vi "소푸틴의 뜻밖의 여정.vi"() -> ()   [LabVIEW 2019]
uses:
  <vilib>/Platform/TimedLoop/XDataNode/timing_clust.ctl
  <vilib>/Platform/TimedLoop/XDataNode/nitl_modes.ctl
  <vilib>/Platform/TimedLoop/XDataNode/wakeup.ctl
  <vilib>/FPGAPlugInAG/myRIO-1900/niLvFpga_Open_myRIO-1900.vi
  <vilib>/rvi/interface/common/dynamic/niFpgaDynamicAddResources.vi
  <vilib>/Utility/error.llb/Error Cluster From Error Code.vi
  <vilib>/rvi/errors/niLvFpgaAdjustHostInterfaceError.vi
  <vilib>/FPGAPlugInAG/Dynamic/niLvFpga_Close_Dynamic.vi
  <vilib>/Platform/TimedLoop/XDataNode/XDataNode.xnode
  <vilib>/rvi/interface/nirviOpenFPGA/nirviOpenFPGA.xnode
  FPGA Bitfiles/untitledproject2_FPGATarget_EncoderPWM(6)2_XV2oDltnHKU.lvbitx
  Encoder_PWM (6).vi
  <vilib>/rvi/interface/nirviReadWriteControl/nirviReadWriteControl.xnode
  <vilib>/rvi/interface/nirviCloseFPGA/nirviCloseFPGA.xnode
  NiFpgaLv.dll
  <vilib>/rvi/interface/Simulation/niFpgaSimulationCallBeginRW.vi
  <vilib>/Platform/TimedLoop/XDataNode/XDNodeRunTimeDep.lvlib
panel:
  out "왼불 5":bool
  out "오른불 4":bool
  out "좌회전":dbl
  out "좌회전":dbl
  out "소푸틴 왼발자취 2":dbl
  out "소푸틴 오른발자취 2":dbl
  in  "stop":bool
  out "왼불 2":bool
  out "오불":bool
  out "소푸틴 왼발자취":dbl
  out "직진 6":dbl
  out "우회전 (30도) 2":dbl
  out "직진 5":dbl
  out "우회전 2":dbl
  out "직진 4":dbl
  out "좌회전 2":dbl
  out "소푸틴 오른발자취":dbl
  in  "초음파":dbl
  in  "잿슨나노":dbl
  out "직진 3":dbl
  out "우회전 (30도)":dbl
  out "직진 2":dbl
  out "우회전":dbl
  out "직진":dbl
  out "좌회전":dbl
  out "Input L 3":dbl[](graph)
  out "Reference & Measurement_L 3":dbl[][](graph)
  in  "Ki 2":dbl
  in  "Kd 2":dbl
  in  "Kp_L":dbl
  out "Input R 2":dbl[](graph)
  out "Reference & Measurement_R 2":dbl[][](graph)
  in  "Ki":dbl
  in  "Kd":dbl
  in  "Kp_R":dbl
  out "u 7":dbl
  out "Mea 4":dbl
  out "Enc_r 2":i32
  out "R_ref":dbl
  out "u 6":dbl
  out "Mea 5":dbl
  out "Enc_r 3":i32
  out "L_ref":dbl
  out "enc":bool
  # "-----------------------------------------------장애물--------------------------------------------------------------"
  # "오른쪽"
  # "왼쪽"
  # "초음파거리 20cm 기준!!"
  # "2200   1700\n\n60    40\n\n\n40   70"
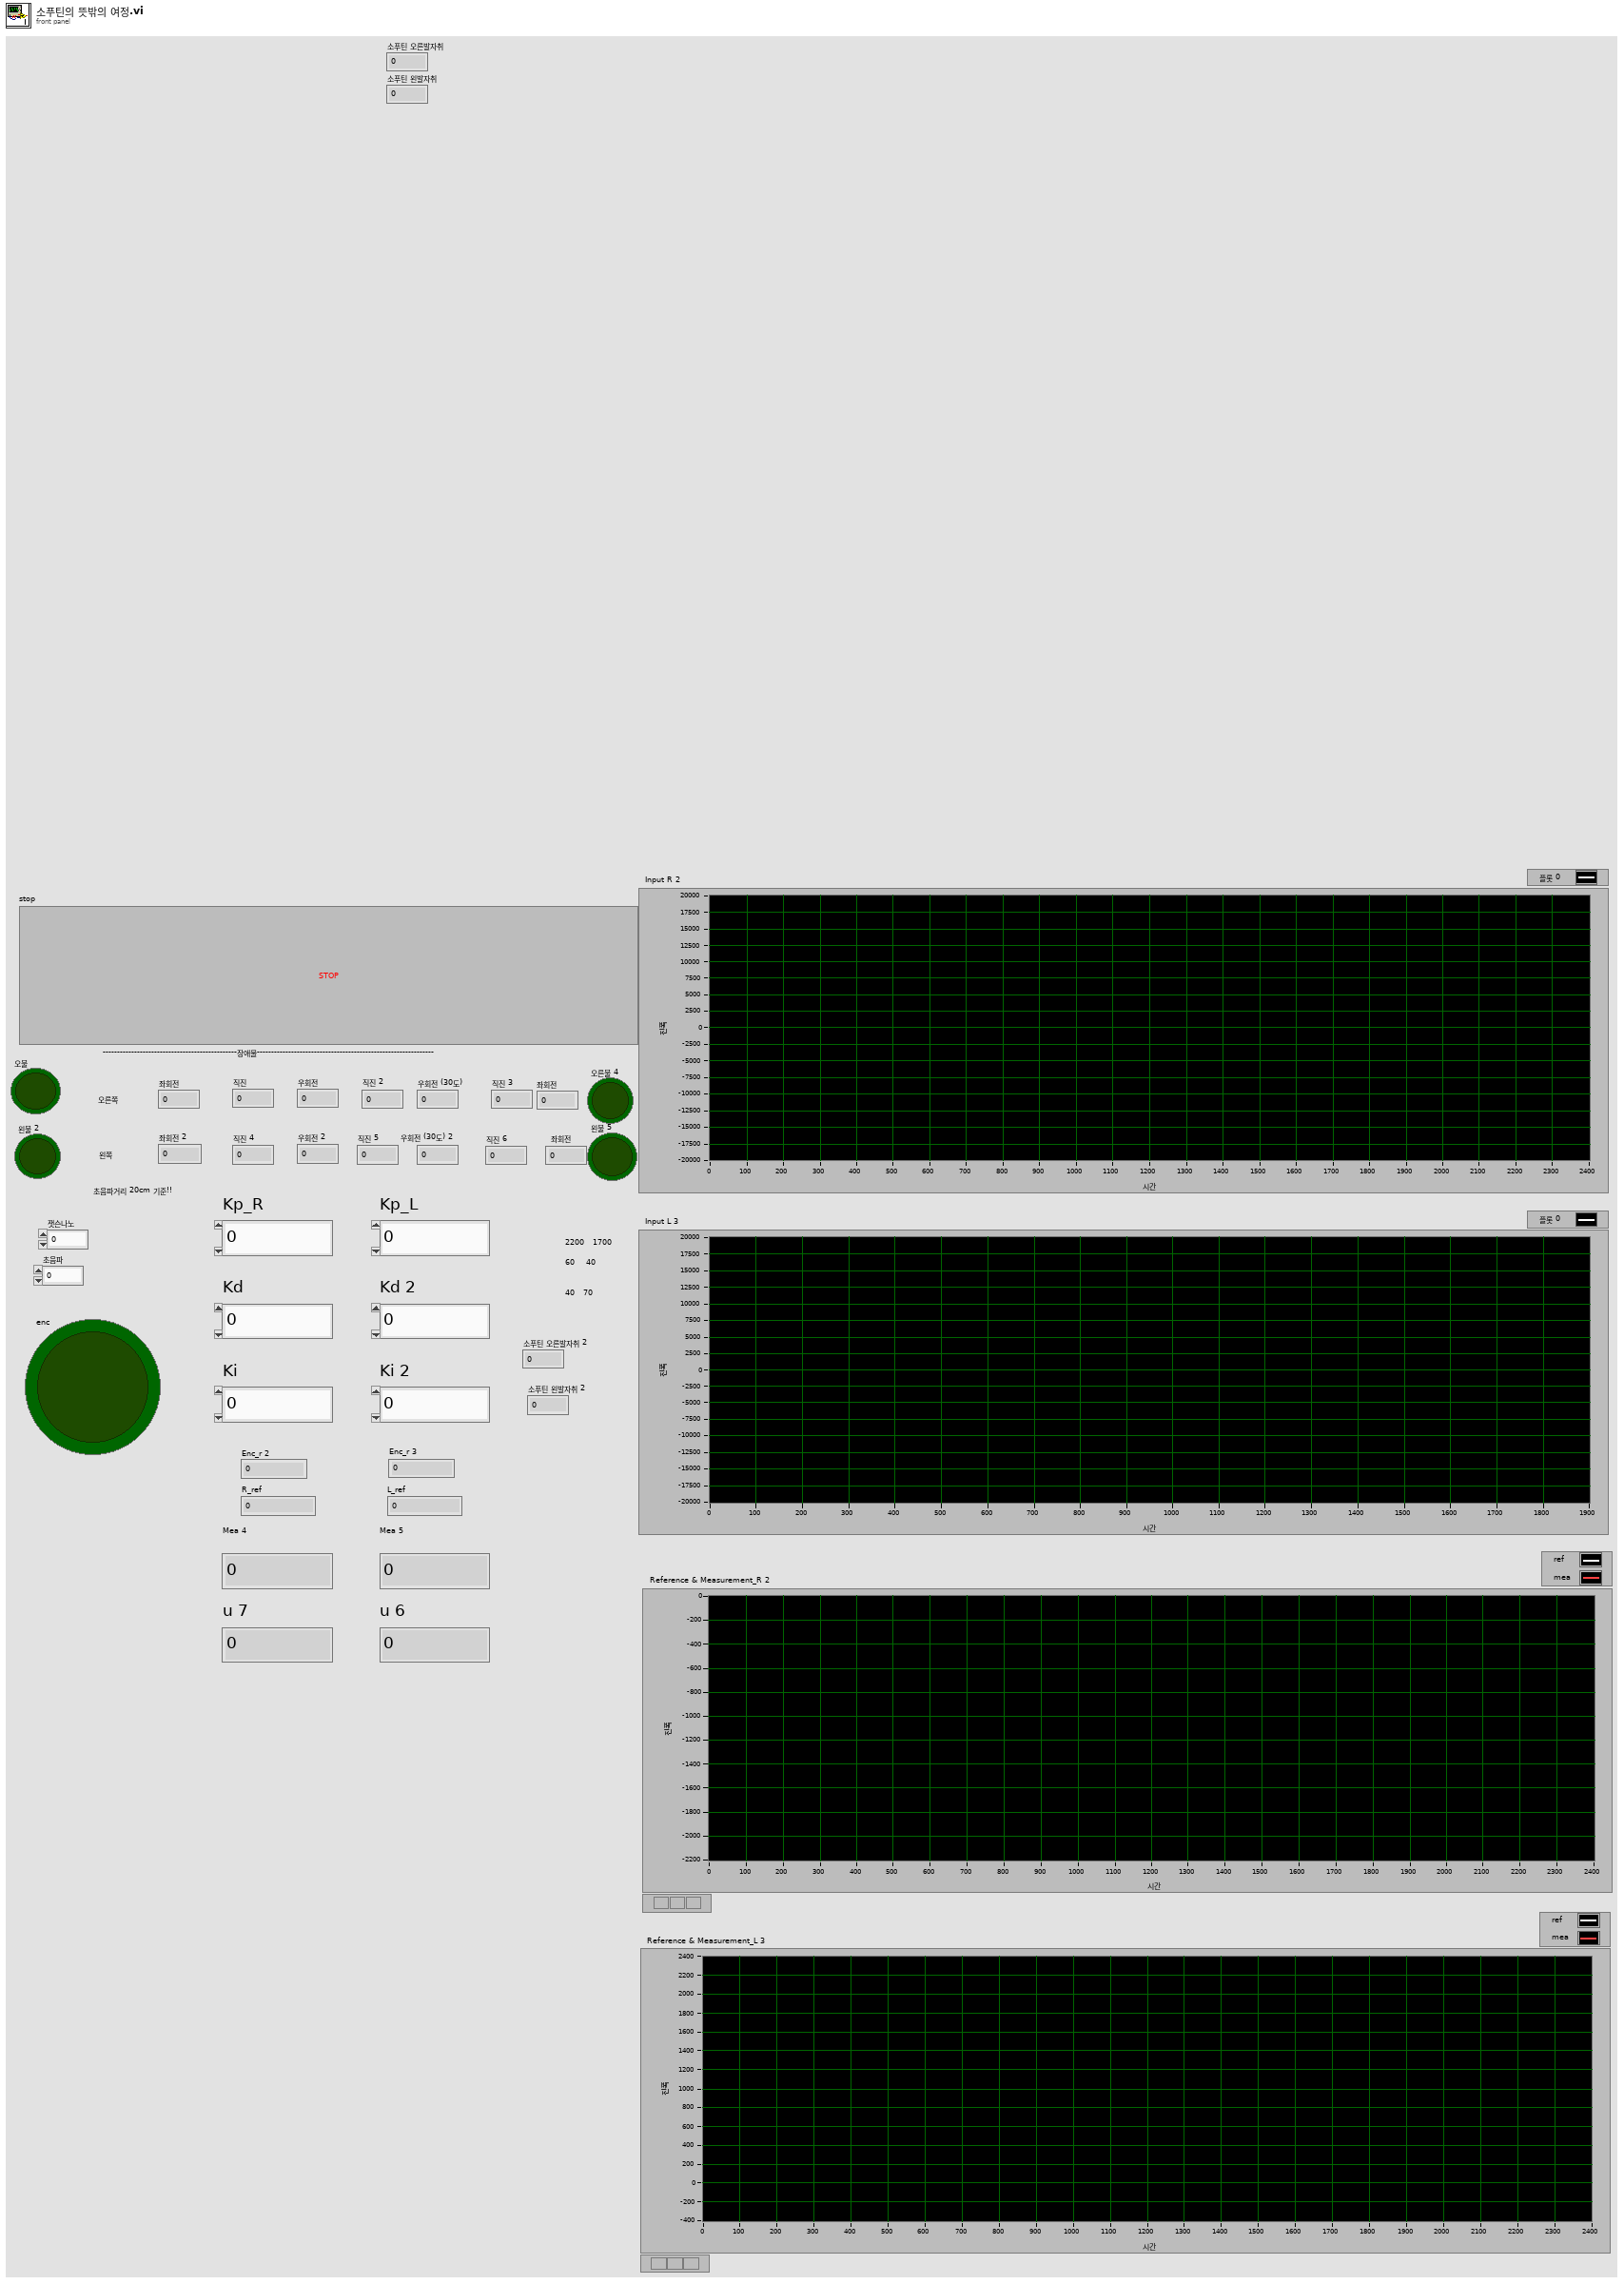
[diagram p1: front panel]
types:
  T1 = typedef "XDNodeRunTimeDep.lvlib/timing_clust.ctl" = cluster{"Expected End [f-1]":u64, "Actual End [f-1]":u64, "Finished Late? [f-1]":bool, "Expected End [i-1]":u64, "Actual End [i-1]":u64, "Finished Late? [i-1]":bool, "Expected Start [i]":u64, "Actual Start [i]":u64, "Expected Start [f]":u64, "Actual Start [f]":u64, "Source Name":string, "Structure Name":string, "Period":i64, "Deadline":i64, "Offset":i64, "Start":i64, "Priority":i32, "Timeout":i32, "Mode":T2, "Wakeup Reason":T3, "Error":errorcluster, "Source Type":string, "Secondary Source Type":string, "Global End Time":u64, "Global Start Time":u64, "Frame Duration":u64, "Iteration Duration":u64, "Assigned CPU":i32, "I/O Scan Engine Mode":u32}
  T2 = typedef "XDNodeRunTimeDep.lvlib/nitl_modes.ctl" = enum32{"No Change", "Process missed periods, maintain original phase", "Discard missed periods, maintain original phase", "Process missed periods, ignore original phase", "Discard missed periods, ignore original phase"}
  T3 = typedef "XDNodeRunTimeDep.lvlib/wakeup.ctl" = enum32{"Normal", "Aborted", "Asynchronous wakeup", "Timing source error", "Timed loop error", "Timeout"}
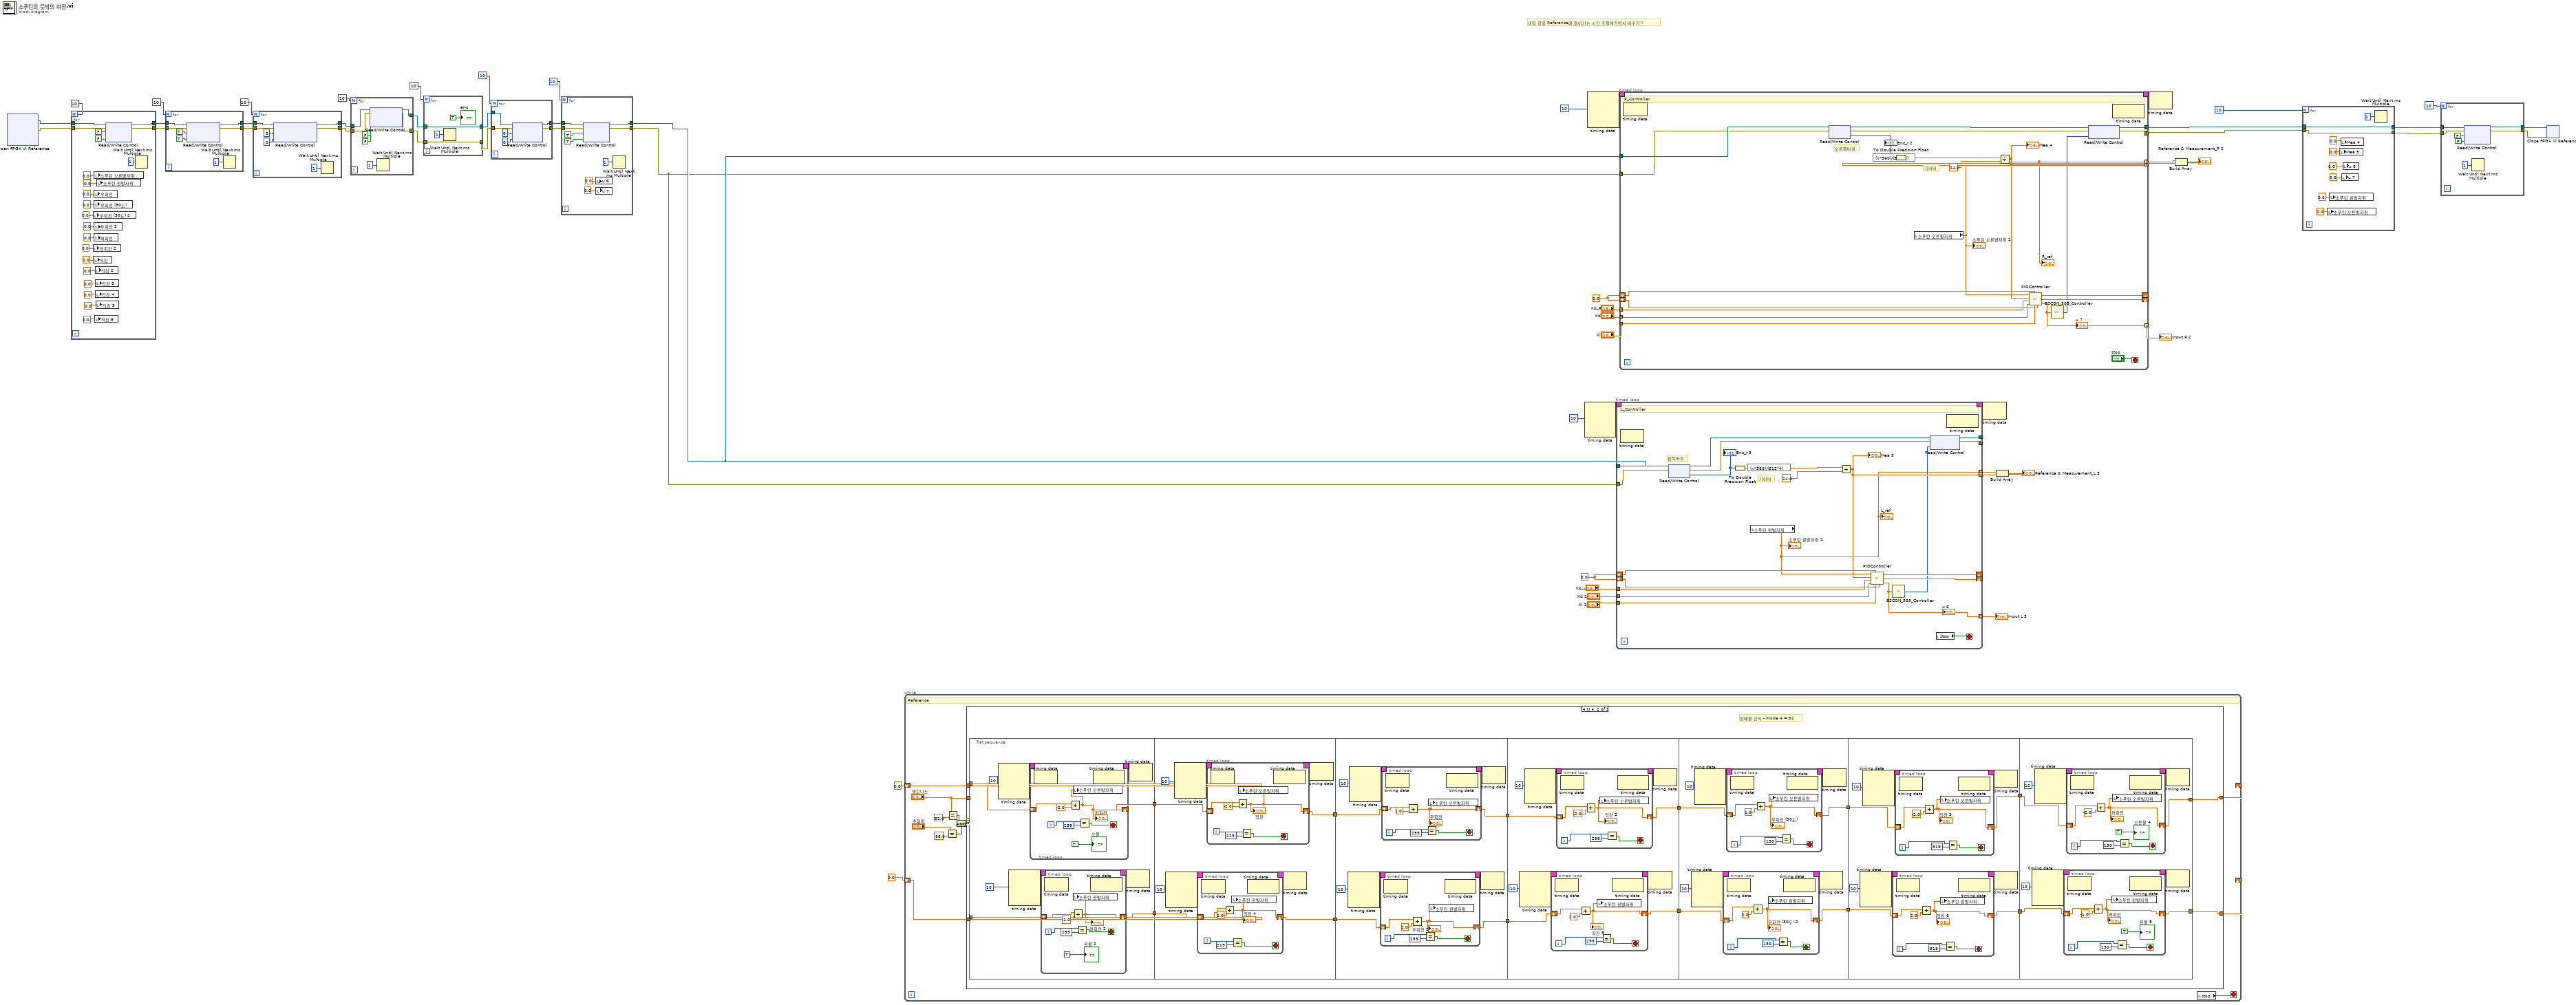
[diagram p0: block diagram]
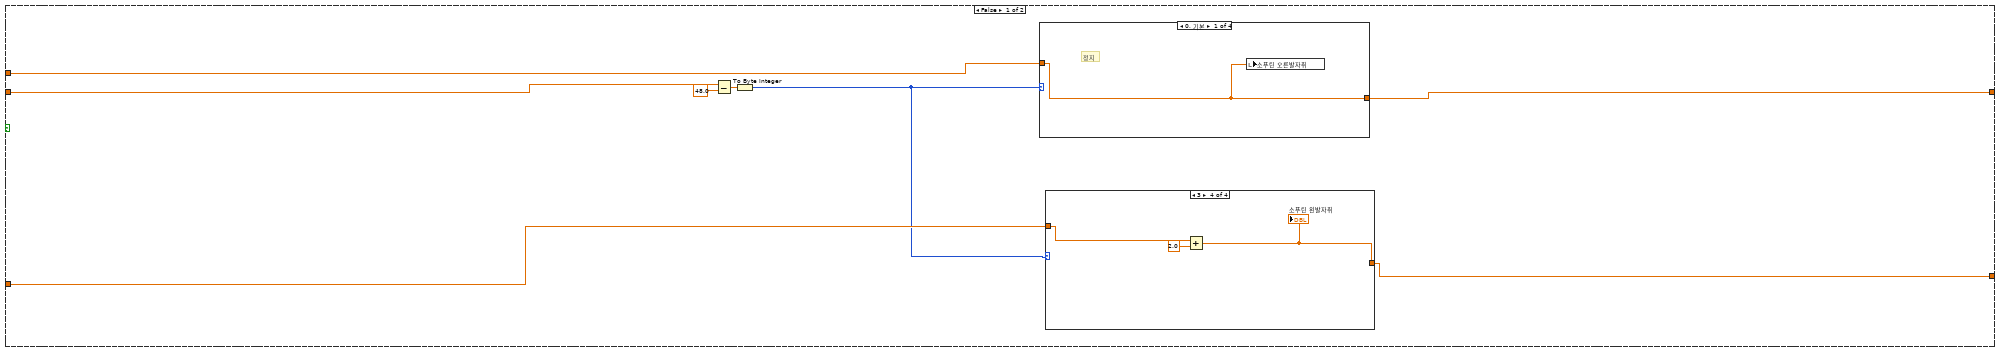
[diagram p2: hidden frame]
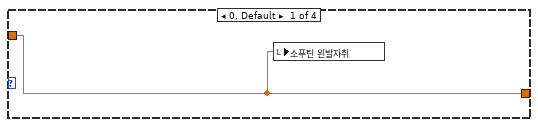
[diagram p3: hidden frame]
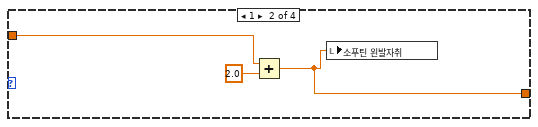
[diagram p4: hidden frame]
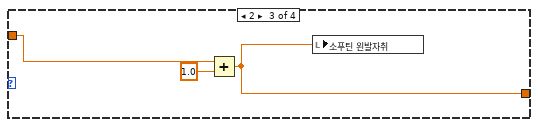
[diagram p5: hidden frame]
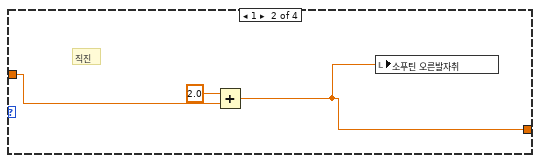
[diagram p6: hidden frame]
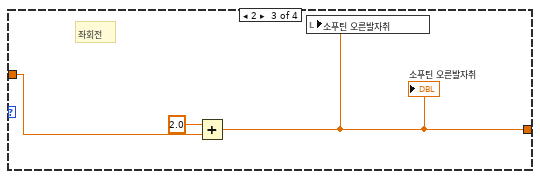
[diagram p7: hidden frame]
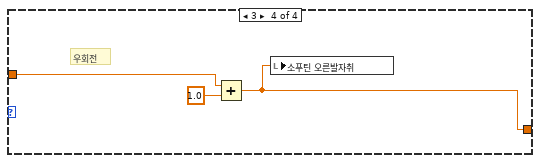
[diagram p8: hidden frame]
diagram:
  w18 = 0.0 ("e")
  w26 = 0.0 ("e")
  # "내일 할일 Reference에 들어가는 시간 조절해가면서 바꾸기!!"
  n1 = xnode "Open FPGA VI Reference"() -> ("FPGA VI 참조 출력"=w36:refnum<k20>, "에러 출력"=w35:errorcluster)  [unwired: 2 in]
  n2 = for {
    N: 10 -> [_]
    tunnel: w36 -> [w75]
    tunnel: w35 -> [w74]
    tunnel: [w73] -> w48
    tunnel: [w72] -> w42
    n3 = local write "우회전 (30도) 2"(0.0 ("우회전 (30도) 2")) -> ()
    n4 = local write "좌회전 2"(0.0 ("좌회전 2")) -> ()
    n5 = local write "직진"(0.0 ("직진")) -> ()
    n6 = local write "우회전"(0.0 ("우회전")) -> ()
    n7 = local write "우회전 (30도)"(0.0 ("우회전 (30도)")) -> ()
    n8 = local write "소푸틴 오른발자취"(0.0) -> ()
    n9 = local write "우회전 2"(0.0 ("우회전 2")) -> ()
    n10 = local write "좌회전"(0.0 ("좌회전")) -> ()
    n11 = local write "직진 6"(0.0 ("직진 6")) -> ()
    n12 = local write "직진 2"(0.0 ("직진 2")) -> ()
    n13 = local write "직진 3"(0.0 ("직진 3")) -> ()
    n14 = local write "직진 4"(0.0 ("직진 4")) -> ()
    n15 = local write "직진 5"(0.0 ("직진 5")) -> ()
    n16 = local write "소푸틴 왼발자취"(0.0) -> ()
    n17 = xnode "Read/Write Control"("FPGA VI 참조 입력"=w75, "에러 입력"=w74, "Enable"=FALSE, "Enable 2"=FALSE) -> ("FPGA VI 참조 출력"=w73:refnum<k20>, "에러 출력"=w72:errorcluster)
    n18 = Wait Until Next ms Multiple(millisecond multiple=u32 1) -> ()  [unwired: 1 out]
  }
  n19 = for {
    N: 10 -> [_]
    tunnel: w48 -> [w81]
    tunnel: [w80] -> w47
    tunnel: w42 -> [w79]
    tunnel: [w78] -> w41
    n20 = xnode "Read/Write Control"("FPGA VI 참조 입력"=w81, "에러 입력"=w79, "Enc_Reset"=TRUE, "Enc_Reset 2"=TRUE) -> ("FPGA VI 참조 출력"=w80:refnum<k20>, "에러 출력"=w78:errorcluster)
    n21 = Wait Until Next ms Multiple(millisecond multiple=u32 1) -> ()  [unwired: 1 out]
  }
  n22 = for {
    N: 10 -> [_]
    tunnel: w47 -> [w89]
    tunnel: [w88] -> w46
    tunnel: w41 -> [w87]
    tunnel: [w86] -> w40
    n23 = xnode "Read/Write Control"("FPGA VI 참조 입력"=w89, "에러 입력"=w87, "Homing Value"=0, "Homing Value 2"=0) -> ("FPGA VI 참조 출력"=w88:refnum<k20>, "에러 출력"=w86:errorcluster)
    n24 = Wait Until Next ms Multiple(millisecond multiple=u32 1) -> ()  [unwired: 1 out]
  }
  n25 = for {
    N: 10 -> [_]
    tunnel: w46 -> [w95]
    tunnel: [w94] -> w45
    tunnel: w40 -> [w93]
    tunnel: [w92] -> w39
    n26 = xnode "Read/Write Control"("FPGA VI 참조 입력"=w95, "에러 입력"=w93, "Enc_Reset"=FALSE, "Enc_Reset 2"=FALSE) -> ("FPGA VI 참조 출력"=w94:refnum<k20>, "에러 출력"=w92:errorcluster)
    n27 = Wait Until Next ms Multiple(millisecond multiple=u32 1) -> ()  [unwired: 1 out]
  }
  n28 = for {
    N: 10 -> [_]
    tunnel: w45 -> [w100]
    tunnel: [w100] -> w44
    tunnel: w39 -> [w99]
    tunnel: [w99] -> w38
    n29 = Wait Until Next ms Multiple(millisecond multiple=u32 1) -> ()  [unwired: 1 out]
    "enc" <- TRUE ("enc")
  }
  n30 = for {
    N: 10 -> [_]
    tunnel: w44 -> [w107]
    tunnel: [w106] -> w43
    tunnel: w38 -> [w105]
    tunnel: [w104] -> w37
    n31 = xnode "Read/Write Control"("FPGA VI 참조 입력"=w107, "에러 입력"=w105, "Input_right"=i16 0, "Input_left"=i16 0) -> ("FPGA VI 참조 출력"=w106:refnum<k20>, "에러 출력"=w104:errorcluster)
  }
  n32 = for {
    N: 10 -> [_]
    tunnel: w43 -> [w114]
    tunnel: w37 -> [w113]
    tunnel: [w111] -> w14
    tunnel: [w110] -> w13
    n33 = xnode "Read/Write Control"("FPGA VI 참조 입력"=w114, "에러 입력"=w113, "Enable"=TRUE, "Enable 2"=TRUE) -> ("FPGA VI 참조 출력"=w111:refnum<k20>, "에러 출력"=w110:errorcluster)
    n34 = local write "u 6"(0.0 ("u 2")) -> ()
    n35 = local write "u 7"(0.0 ("u")) -> ()
    n36 = Wait Until Next ms Multiple(millisecond multiple=u32 1) -> ()  [unwired: 1 out]
  }
  n37 = while {
    shift-right: [w120] -> _
    shift-left: 0.0 -> [w121]
    shift-right: [w118] -> _
    shift-left: 0.0 -> [w119]
    stop <- w117 stop-if-true
    # "Reference"
    n38 = Equal?(x="초음파", y=96.0) -> (x = y?=w125:bool)
    n39 = Equal?(x="잿슨나노", y=52.0) -> (x = y?=w127:bool)
    n40 = And(x=w127, y=w125) -> (x .and. y?=w124:bool)
    n41 = case shown="참" w124 {
      tunnel: "잿슨나노" -> [w134 _]
      tunnel: w121 -> [w136 w172]
      tunnel: [w135 w157] -> w120
      tunnel: w119 -> [w131 w166]
      tunnel: [w129 w158] -> w118
      frame False {
        n42 = Subtract(x=w134, y=48.0) -> (x-y=w132:dbl)
        n43 = To Byte Integer(number=w132) -> (8bit integer=w130:i8)
        n44 = case shown="0, 기본" w130 {
          tunnel: w136 -> [w147 w150 w153 w155]
          tunnel: [w147 w148 w151 w156] -> w135
          frame 0, Default {
            # "정지"
            n45 = local write "소푸틴 오른발자취"(w147) -> ()
          }
          frame 1 {
            # "직진"
            n46 = Add(x=2.0, y=w150) -> (x+y=w148:dbl)
            n47 = local write "소푸틴 오른발자취"(w148) -> ()
          }
          frame 2 {
            # "좌회전"
            n48 = Add(x=2.0, y=w153) -> (x+y=w151:dbl)
            "소푸틴 오른발자취" <- w151
            n49 = local write "소푸틴 오른발자취"(w151) -> ()
          }
          frame 3 {
            # "우회전"
            n50 = Add(x=w155, y=1.0) -> (x+y=w156:dbl)
            n51 = local write "소푸틴 오른발자취"(w156) -> ()
          }
        }
        n52 = case shown="3" w130 {
          tunnel: w131 -> [w137 w139 w143 w146]
          tunnel: [w137 w140 w141 w144] -> w129
          frame 0, Default {
            n53 = local write "소푸틴 왼발자취"(w137) -> ()
          }
          frame 1 {
            n54 = Add(x=w139, y=2.0) -> (x+y=w140:dbl)
            n55 = local write "소푸틴 왼발자취"(w140) -> ()
          }
          frame 2 {
            n56 = Add(x=w143, y=1.0) -> (x+y=w141:dbl)
            n57 = local write "소푸틴 왼발자취"(w141) -> ()
          }
          frame 3 {
            n58 = Add(x=w146, y=2.0) -> (x+y=w144:dbl)
            "소푸틴 왼발자취" <- w144
          }
        }
      }
      frame True {
        # "장애물 인식 - mode 4 = 52"
        n59 = flat-sequence {
          tunnel: w172 -> [w175]
          tunnel: [w179] -> w171
          tunnel: w166 -> [w174]
          tunnel: [w173] -> w165
          tunnel: w171 -> [w212]
          tunnel: [w211] -> w170
          tunnel: w165 -> [w210]
          tunnel: [w209] -> w164
          tunnel: w170 -> [w246]
          tunnel: [w245] -> w169
          tunnel: w164 -> [w244]
          tunnel: [w243] -> w163
          tunnel: w169 -> [w280]
          tunnel: [w279] -> w168
          tunnel: w163 -> [w278]
          tunnel: [w277] -> w162
          tunnel: w168 -> [w314]
          tunnel: [w313] -> w167
          tunnel: w162 -> [w312]
          tunnel: [w311] -> w161
          tunnel: w167 -> [w348]
          tunnel: w161 -> [w346]
          tunnel: [w345] -> w160
          tunnel: [w347] -> w159
          tunnel: w160 -> [w381]
          tunnel: w159 -> [w382]
          tunnel: [w380] -> w158
          tunnel: [w379] -> w157
          frame #0 {
            n60 = node-c288(i64 10 ("Period")) -> (w182:T1)  [unwired: 3 in]
            n61 = node-c288(i64 10 ("Period")) -> (w178:T1)  [unwired: 3 in]
            n62 = timed-loop {
              timing: w182 -> [_]
              timing-out: [_] -> w181
              shift-right: [w198] -> w179
              shift-left: w175 -> [w197]
              i -> [w201]
              stop <- w200 stop-if-true
              n63 = node-c288() -> ()  [unwired: 1 in, 1 out]
              n64 = Add(x=w197, y=-2.0) -> (x+y=w198:dbl)
              "좌회전" <- w198
              n65 = local write "소푸틴 오른발자취"(w198) -> ()
              n66 = Equal?(x=w201, y=259) -> (x = y?=w200:bool)
              n67 = node-c288() -> ()  [unwired: 1 in, 1 out]
              "오불" <- TRUE
            }
            n68 = timed-loop {
              timing: w178 -> [_]
              timing-out: [_] -> w177
              shift-right: [w183] -> w173
              shift-left: w174 -> [w184]
              i -> [w187]
              stop <- w186 stop-if-true
              n69 = node-c288() -> ()  [unwired: 1 in, 1 out]
              n70 = Add(x=w184, y=-1.0) -> (x+y=w183:dbl)
              "좌회전 2" <- w183
              n71 = local write "소푸틴 왼발자취"(w183) -> ()
              n72 = Equal?(x=w187, y=259) -> (x = y?=w186:bool)
              n73 = node-c288() -> ()  [unwired: 1 in, 1 out]
              "왼불 2" <- TRUE
            }
            n74 = node-c288(w177) -> ()  [unwired: 1 out]
            n75 = node-c288(w181) -> ()  [unwired: 1 out]
          }
          frame #1 {
            n76 = node-c288(i64 10 ("Period")) -> (w215:T1)  [unwired: 3 in]
            n77 = node-c288(i64 10 ("Period")) -> (w218:T1)  [unwired: 3 in]
            n78 = timed-loop {
              timing: w215 -> [_]
              timing-out: [_] -> w214
              shift-right: [w219] -> w209
              shift-left: w210 -> [w220]
              i -> [w223]
              stop <- w221 stop-if-true
              n79 = node-c288() -> ()  [unwired: 1 in, 1 out]
              n80 = Add(x=w220, y=2.0) -> (x+y=w219:dbl)
              "직진 4" <- w219
              n81 = Equal?(x=w223, y=219) -> (x = y?=w221:bool)
              n82 = local write "소푸틴 왼발자취"(w219) -> ()
              n83 = node-c288() -> ()  [unwired: 1 in, 1 out]
            }
            n84 = timed-loop {
              timing: w218 -> [_]
              timing-out: [_] -> w217
              shift-right: [w233] -> w211
              shift-left: w212 -> [w232]
              i -> [w236]
              stop <- w234 stop-if-true
              n85 = node-c288() -> ()  [unwired: 1 in, 1 out]
              n86 = Add(x=w232, y=-2.0) -> (x+y=w233:dbl)
              "직진" <- w233
              n87 = local write "소푸틴 오른발자취"(w233) -> ()
              n88 = Equal?(x=w236, y=219) -> (x = y?=w234:bool)
              n89 = node-c288() -> ()  [unwired: 1 in, 1 out]
            }
            n90 = node-c288(w214) -> ()  [unwired: 1 out]
            n91 = node-c288(w217) -> ()  [unwired: 1 out]
          }
          frame #2 {
            n92 = node-c288(i64 10 ("Period")) -> (w249:T1)  [unwired: 3 in]
            n93 = node-c288(i64 10 ("Period")) -> (w252:T1)  [unwired: 3 in]
            n94 = timed-loop {
              timing: w249 -> [_]
              timing-out: [_] -> w248
              shift-right: [w254] -> w243
              shift-left: w244 -> [w253]
              i -> [w256]
              stop <- w255 stop-if-true
              n95 = node-c288() -> ()  [unwired: 1 in, 1 out]
              n96 = Add(x=w253, y=2.0) -> (x+y=w254:dbl)
              "우회전 2" <- w254
              n97 = Equal?(x=w256, y=259) -> (x = y?=w255:bool)
              n98 = local write "소푸틴 왼발자취"(w254) -> ()
              n99 = node-c288() -> ()  [unwired: 1 in, 1 out]
            }
            n100 = timed-loop {
              timing: w252 -> [_]
              timing-out: [_] -> w251
              shift-right: [w267] -> w245
              shift-left: w246 -> [w266]
              i -> [w269]
              stop <- w268 stop-if-true
              n101 = node-c288() -> ()  [unwired: 1 in, 1 out]
              n102 = Add(x=w266, y=1.0) -> (x+y=w267:dbl)
              "우회전" <- w267
              n103 = Equal?(x=w269, y=259) -> (x = y?=w268:bool)
              n104 = local write "소푸틴 오른발자취"(w267) -> ()
              n105 = node-c288() -> ()  [unwired: 1 in, 1 out]
            }
            n106 = node-c288(w248) -> ()  [unwired: 1 out]
            n107 = node-c288(w251) -> ()  [unwired: 1 out]
          }
          frame #3 {
            n108 = node-c288(i64 10 ("Period")) -> (w283:T1)  [unwired: 3 in]
            n109 = node-c288(i64 10 ("Period")) -> (w286:T1)  [unwired: 3 in]
            n110 = timed-loop {
              timing: w283 -> [_]
              timing-out: [_] -> w282
              shift-right: [w287] -> w277
              shift-left: w278 -> [w288]
              i -> [w290]
              stop <- w289 stop-if-true
              n111 = node-c288() -> ()  [unwired: 1 in, 1 out]
              n112 = Add(x=w288, y=2.0) -> (x+y=w287:dbl)
              "직진 5" <- w287
              n113 = local write "소푸틴 왼발자취"(w287) -> ()
              n114 = Equal?(x=w290, y=299) -> (x = y?=w289:bool)
              n115 = node-c288() -> ()  [unwired: 1 in, 1 out]
            }
            n116 = timed-loop {
              timing: w286 -> [_]
              timing-out: [_] -> w285
              shift-right: [w299] -> w279
              shift-left: w280 -> [w300]
              i -> [w302]
              stop <- w301 stop-if-true
              n117 = node-c288() -> ()  [unwired: 1 in, 1 out]
              n118 = Add(x=w300, y=-2.0) -> (x+y=w299:dbl)
              "직진 2" <- w299
              n119 = local write "소푸틴 오른발자취"(w299) -> ()
              n120 = Equal?(x=w302, y=299) -> (x = y?=w301:bool)
              n121 = node-c288() -> ()  [unwired: 1 in, 1 out]
            }
            n122 = node-c288(w282) -> ()  [unwired: 1 out]
            n123 = node-c288(w285) -> ()  [unwired: 1 out]
          }
          frame #4 {
            n124 = node-c288(i64 10 ("Period")) -> (w317:T1)  [unwired: 3 in]
            n125 = node-c288(i64 10 ("Period")) -> (w320:T1)  [unwired: 3 in]
            n126 = timed-loop {
              timing: w317 -> [_]
              timing-out: [_] -> w316
              shift-right: [w321] -> w311
              shift-left: w312 -> [w322]
              i -> [w324]
              stop <- w323 stop-if-true
              n127 = node-c288() -> ()  [unwired: 1 in, 1 out]
              n128 = Add(x=w322, y=2.0) -> (x+y=w321:dbl)
              "우회전 (30도) 2" <- w321
              n129 = local write "소푸틴 왼발자취"(w321) -> ()
              n130 = Equal?(x=w324, y=150) -> (x = y?=w323:bool)
              n131 = node-c288() -> ()  [unwired: 1 in, 1 out]
            }
            n132 = timed-loop {
              timing: w320 -> [_]
              timing-out: [_] -> w319
              shift-right: [w334] -> w313
              shift-left: w314 -> [w333]
              i -> [w336]
              stop <- w335 stop-if-true
              n133 = node-c288() -> ()  [unwired: 1 in, 1 out]
              n134 = Add(x=w333, y=1.0) -> (x+y=w334:dbl)
              "우회전 (30도)" <- w334
              n135 = local write "소푸틴 오른발자취"(w334) -> ()
              n136 = Equal?(x=w336, y=150) -> (x = y?=w335:bool)
              n137 = node-c288() -> ()  [unwired: 1 in, 1 out]
            }
            n138 = node-c288(w316) -> ()  [unwired: 1 out]
            n139 = node-c288(w319) -> ()  [unwired: 1 out]
          }
          frame #5 {
            n140 = node-c288(i64 10 ("Period")) -> (w351:T1)  [unwired: 3 in]
            n141 = node-c288(i64 10 ("Period")) -> (w354:T1)  [unwired: 3 in]
            n142 = timed-loop {
              timing: w351 -> [_]
              timing-out: [_] -> w350
              shift-right: [w355] -> w345
              shift-left: w346 -> [w356]
              i -> [w358]
              stop <- w357 stop-if-true
              n143 = node-c288() -> ()  [unwired: 1 in, 1 out]
              n144 = Add(x=w356, y=2.0) -> (x+y=w355:dbl)
              "직진 6" <- w355
              n145 = local write "소푸틴 왼발자취"(w355) -> ()
              n146 = Equal?(x=w358, y=319) -> (x = y?=w357:bool)
              n147 = node-c288() -> ()  [unwired: 1 in, 1 out]
            }
            n148 = timed-loop {
              timing: w354 -> [_]
              timing-out: [_] -> w353
              shift-right: [w367] -> w347
              shift-left: w348 -> [w368]
              i -> [w370]
              stop <- w369 stop-if-true
              n149 = node-c288() -> ()  [unwired: 1 in, 1 out]
              n150 = Add(x=w368, y=-2.0) -> (x+y=w367:dbl)
              "직진 3" <- w367
              n151 = local write "소푸틴 오른발자취"(w367) -> ()
              n152 = Equal?(x=w370, y=319) -> (x = y?=w369:bool)
              n153 = node-c288() -> ()  [unwired: 1 in, 1 out]
            }
            n154 = node-c288(w353) -> ()  [unwired: 1 out]
            n155 = node-c288(w350) -> ()  [unwired: 1 out]
          }
          frame #6 {
            n156 = node-c288(i64 10 ("Period")) -> (w386:T1)  [unwired: 3 in]
            n157 = node-c288(i64 10 ("Period")) -> (w388:T1)  [unwired: 3 in]
            n158 = timed-loop {
              timing: w386 -> [_]
              timing-out: [_] -> w385
              shift-right: [w390] -> w380
              shift-left: w381 -> [w391]
              i -> [w393]
              stop <- w392 stop-if-true
              n159 = node-c288() -> ()  [unwired: 1 in, 1 out]
              n160 = Add(x=w391, y=-1.0) -> (x+y=w390:dbl)
              "좌회전" <- w390
              n161 = local write "소푸틴 왼발자취"(w390) -> ()
              n162 = Equal?(x=w393, y=150) -> (x = y?=w392:bool)
              n163 = node-c288() -> ()  [unwired: 1 in, 1 out]
              "왼불 5" <- TRUE
            }
            n164 = timed-loop {
              timing: w388 -> [_]
              timing-out: [_] -> w387
              shift-right: [w403] -> w379
              shift-left: w382 -> [w404]
              i -> [w406]
              stop <- w405 stop-if-true
              n165 = node-c288() -> ()  [unwired: 1 in, 1 out]
              n166 = Add(x=w404, y=-2.0) -> (x+y=w403:dbl)
              "좌회전" <- w403
              n167 = local write "소푸틴 오른발자취"(w403) -> ()
              n168 = Equal?(x=w406, y=150) -> (x = y?=w405:bool)
              n169 = node-c288() -> ()  [unwired: 1 in, 1 out]
              "오른불 4" <- TRUE
            }
            n170 = node-c288(w387) -> ()  [unwired: 1 out]
            n171 = node-c288(w385) -> ()  [unwired: 1 out]
          }
        }
      }
    }
    n172 = local read "stop"() -> (w117:bool)
  }
  n173 = node-c288(i64 10 ("주기")) -> (w34:T1)  [unwired: 3 in]
  n174 = node-c288(i64 10 ("주기")) -> (w32:T1)  [unwired: 3 in]
  n175 = timed-loop {
    timing: w34 -> [_]
    timing-out: [_] -> w33
    tunnel: "Kp_L" -> [w427]
    tunnel: "Kd 2" -> [w428]
    tunnel: "Ki 2" -> [w429]
    shift-right: [w432] -> _
    shift-left: w18 -> [w433]
    shift-right: [w431] -> _
    shift-left: w18 -> [w425]
    tunnel: [w426] -> w16 mode=indexing
    tunnel: [w430] -> w15 mode=indexing
    tunnel: [w422] -> _
    tunnel: [w421] -> _
    tunnel: w14 -> [w420]
    tunnel: w13 -> [w417]
    tunnel: [w416] -> w2 mode=indexing
    stop <- w415 stop-if-true
    # "왼쪽바퀴"
    # "기어비"
    # "L_Controller"
    n176 = node-c288() -> ()  [unwired: 1 in, 1 out]
    n177 = xnode "Read/Write Control"("FPGA VI 참조 입력"=w420, "에러 입력"=w417) -> ("FPGA VI 참조 출력"=w424:refnum<k20>, "에러 출력"=w423:errorcluster, "Enc 2"=w418:i32)
    "Enc_r 3" <- w418
    n178 = To Double Precision Float(number=w418) -> (double precision float=w434:dbl)
    n179 = expression code="(x*360)/(512*4)"(w434) -> (w436:dbl)
    n180 = local read "소푸틴 왼발자취"() -> (w416:dbl)
    "L_ref" <- w416
    "소푸틴 왼발자취 2" <- w416
    n181 = Divide(x=w436, y=24.0) -> (x/y=w426:dbl)
    "Mea 5" <- w426
    n182 = call "PIDController.vi"("e_Sum_Old"=w425, "Ki"=w429, "Kd"=w428, "Kp"=w427, "eOld"=w433, "Measurement"=w426, "Reference"=w416) -> ("u"=w430:dbl, "e_Sum"=w431:dbl, "e"=w432:dbl)  [unwired: 1 in]
    "u 6" <- w430
    n183 = call "ESCON_505_Controller.vi"("u"=w430) -> ("Modified u"=w419:i16)
    n184 = xnode "Read/Write Control"("FPGA VI 참조 입력"=w424, "에러 입력"=w423, "Input_left"=w419) -> ("FPGA VI 참조 출력"=w422:refnum<k20>, "에러 출력"=w421:errorcluster)
    n185 = local read "stop"() -> (w415:bool)
    n186 = node-c288() -> ()  [unwired: 1 in, 1 out]
  }
  "Input L 3" <- w15
  n187 = timed-loop {
    timing: w32 -> [_]
    timing-out: [_] -> w31
    tunnel: "Kp_R" -> [w451]
    tunnel: "Kd" -> [w452]
    tunnel: "Ki" -> [w453]
    shift-right: [w456] -> _
    shift-left: w26 -> [w457]
    shift-right: [w455] -> _
    shift-left: w26 -> [w449]
    tunnel: [w450] -> w24 mode=indexing
    tunnel: [w454] -> w23 mode=indexing
    tunnel: [w446] -> w6
    tunnel: [w445] -> w5
    tunnel: w14 -> [w444]
    tunnel: w13 -> [w441]
    tunnel: [w440] -> w1 mode=indexing
    stop <- "stop" stop-if-true
    # "오른쪽바퀴"
    # "기어비"
    # "R_Controller"
    n188 = node-c288() -> ()  [unwired: 1 in, 1 out]
    n189 = xnode "Read/Write Control"("FPGA VI 참조 입력"=w444, "에러 입력"=w441) -> ("FPGA VI 참조 출력"=w448:refnum<k20>, "에러 출력"=w447:errorcluster, "Enc"=w442:i32)
    "Enc_r 2" <- w442
    n190 = To Double Precision Float(number=w442) -> (double precision float=w458:dbl)
    n191 = expression code="(x*360)/(512*4)"(w458) -> (w460:dbl)
    n192 = local read "소푸틴 오른발자취"() -> (w440:dbl)
    "R_ref" <- w440
    "소푸틴 오른발자취 2" <- w440
    n193 = Divide(x=w460, y=24.0) -> (x/y=w450:dbl)
    "Mea 4" <- w450
    n194 = call "PIDController.vi"("e_Sum_Old"=w449, "Ki"=w453, "Kd"=w452, "Kp"=w451, "eOld"=w457, "Measurement"=w450, "Reference"=w440) -> ("u"=w454:dbl, "e_Sum"=w455:dbl, "e"=w456:dbl)  [unwired: 1 in]
    "u 7" <- w454
    n195 = call "ESCON_505_Controller.vi"("u"=w454) -> ("Modified u"=w443:i16)
    n196 = xnode "Read/Write Control"("FPGA VI 참조 입력"=w448, "에러 입력"=w447, "Input_right"=w443) -> ("FPGA VI 참조 출력"=w446:refnum<k20>, "에러 출력"=w445:errorcluster)
    n197 = node-c288() -> ()  [unwired: 1 in, 1 out]
  }
  "Input R 2" <- w23
  n198 = node-c288(w33) -> ()  [unwired: 1 out]
  n199 = Build Array(w2, w16) -> (→"Reference & Measurement_L 3":dbl[][])
  n200 = node-c288(w31) -> ()  [unwired: 1 out]
  n201 = Build Array(w1, w24) -> (→"Reference & Measurement_R 2":dbl[][])
  n202 = for {
    N: 10 -> [_]
    tunnel: [w470] -> w8
    tunnel: w6 -> [w470]
    tunnel: w5 -> [w469]
    tunnel: [w469] -> w9
    n203 = local write "소푸틴 오른발자취"(0.0 ("소푸틴 오른발자취")) -> ()
    n204 = local write "소푸틴 왼발자취"(0.0 ("소푸틴 왼발자취")) -> ()
    n205 = local write "Mea 5"(0.0 ("Mea 2")) -> ()
    n206 = local write "Mea 4"(0.0 ("Mea")) -> ()
    n207 = local write "u 7"(0.0 ("u")) -> ()
    n208 = local write "u 6"(0.0 ("Mea 3")) -> ()
    n209 = Wait Until Next ms Multiple(millisecond multiple=u32 1) -> ()  [unwired: 1 out]
  }
  n210 = for {
    N: 10 -> [_]
    tunnel: w8 -> [w478]
    tunnel: w9 -> [w477]
    tunnel: [w473] -> w11
    tunnel: [w472] -> w12
    n211 = xnode "Read/Write Control"("FPGA VI 참조 입력"=w478, "에러 입력"=w477, "Enable"=FALSE, "Enable 2"=FALSE) -> ("FPGA VI 참조 출력"=w473:refnum<k20>, "에러 출력"=w472:errorcluster)
    n212 = Wait Until Next ms Multiple(millisecond multiple=u32 1) -> ()  [unwired: 1 out]
  }
  n213 = xnode "Close FPGA VI Reference"("FPGA VI Reference In"=w11, "error in"=w12) -> ()  [unwired: 1 out]
